vi "test4-MacroWithNonLocalSubMessages.vi"(8 "error in":errorcluster, 11 "TestCase in":refnum<class "testcase-CSMResponse.lvclass">) -> (0 "error out":errorcluster, 3 "TestCase out":refnum<class "testcase-CSMResponse.lvclass">)   [LabVIEW 2017, in "testcase-CSMResponse.lvclass"]
uses:
  testcase-CSMResponse.lvclass
  0c6454a9-3719-4e31-9ff6-45b39d38beb6.vi
  2437fcdf-222d-44ea-9250-34e015767128.vi
  src/user.lib/_NEVSTOP/Communicable State Machine(CSM)/AdvanceAPI/CSM - Get Module Attribute.vi
  <vilib>/addons/_JKI Toolkits/VI Tester/TestCase.llb/TestCase.lvclass
  src/user.lib/_NEVSTOP/Communicable State Machine(CSM)/Communicable State Machine.lvlib
  C:/Program Files (x86)/National Instruments/LabVIEW 2017/vi.lib/addons/_JKI Toolkits/VI Tester/TestCase.llb/TestCase.lvclass
panel:
  out "Loopcount":i32
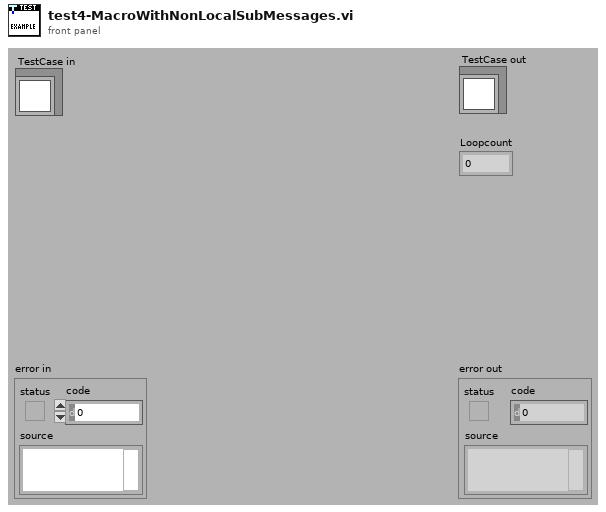
[diagram p1: front panel]
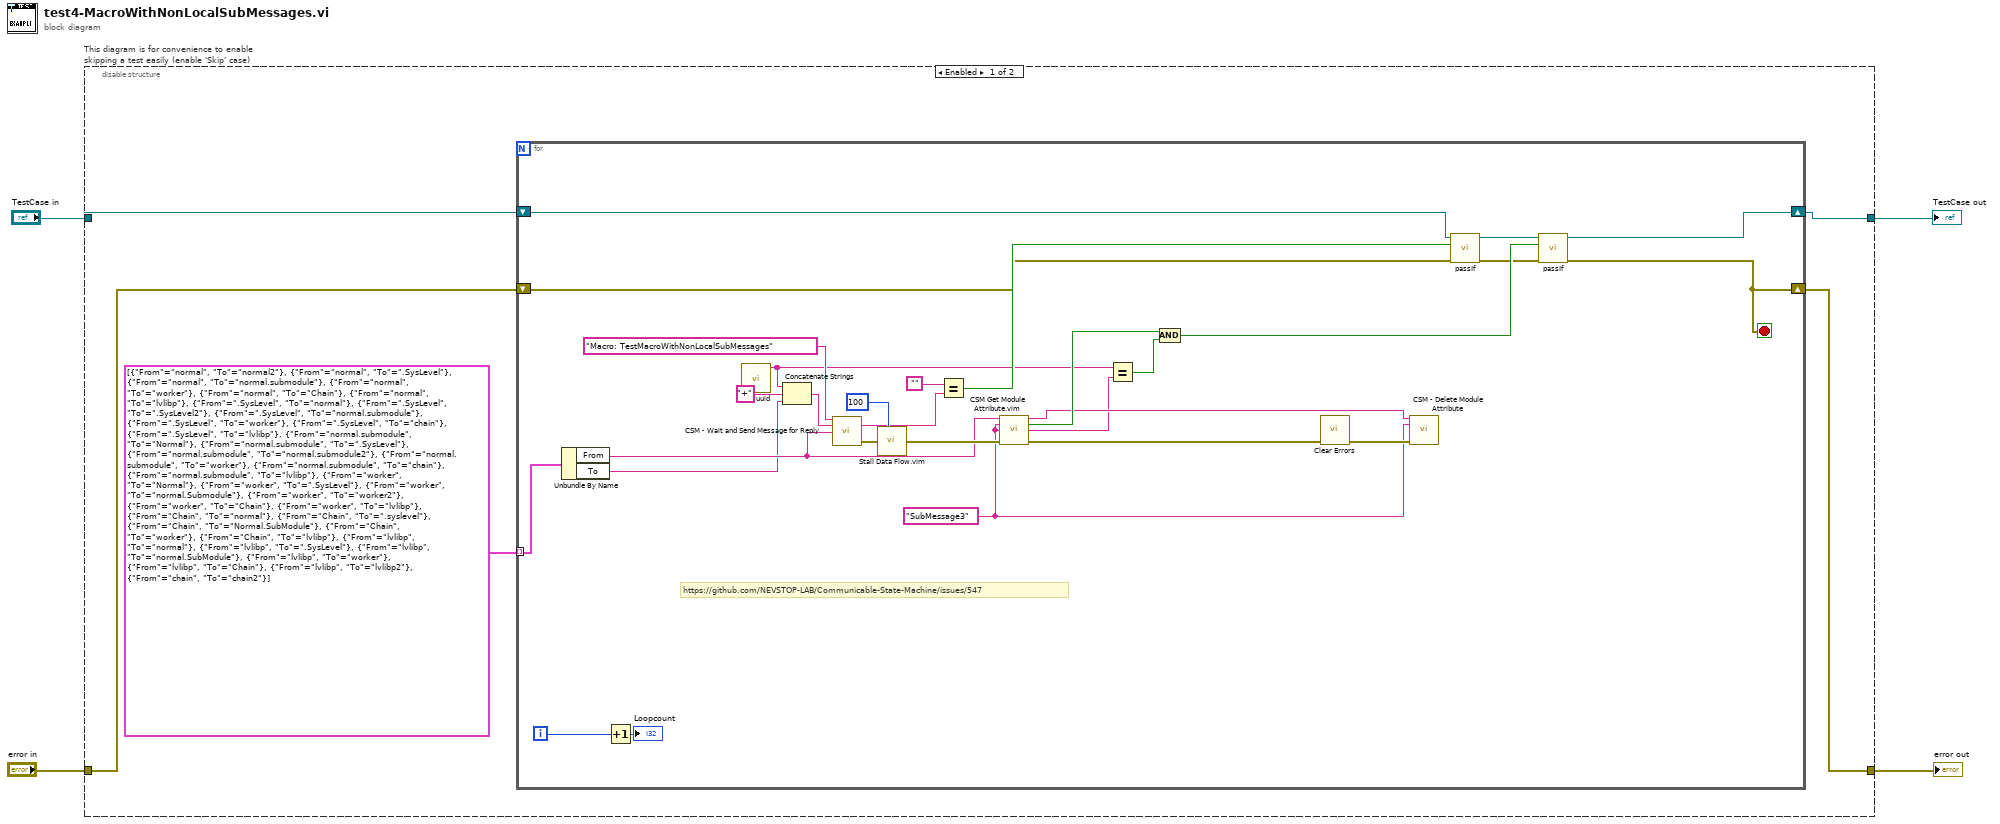
[diagram p0: block diagram]
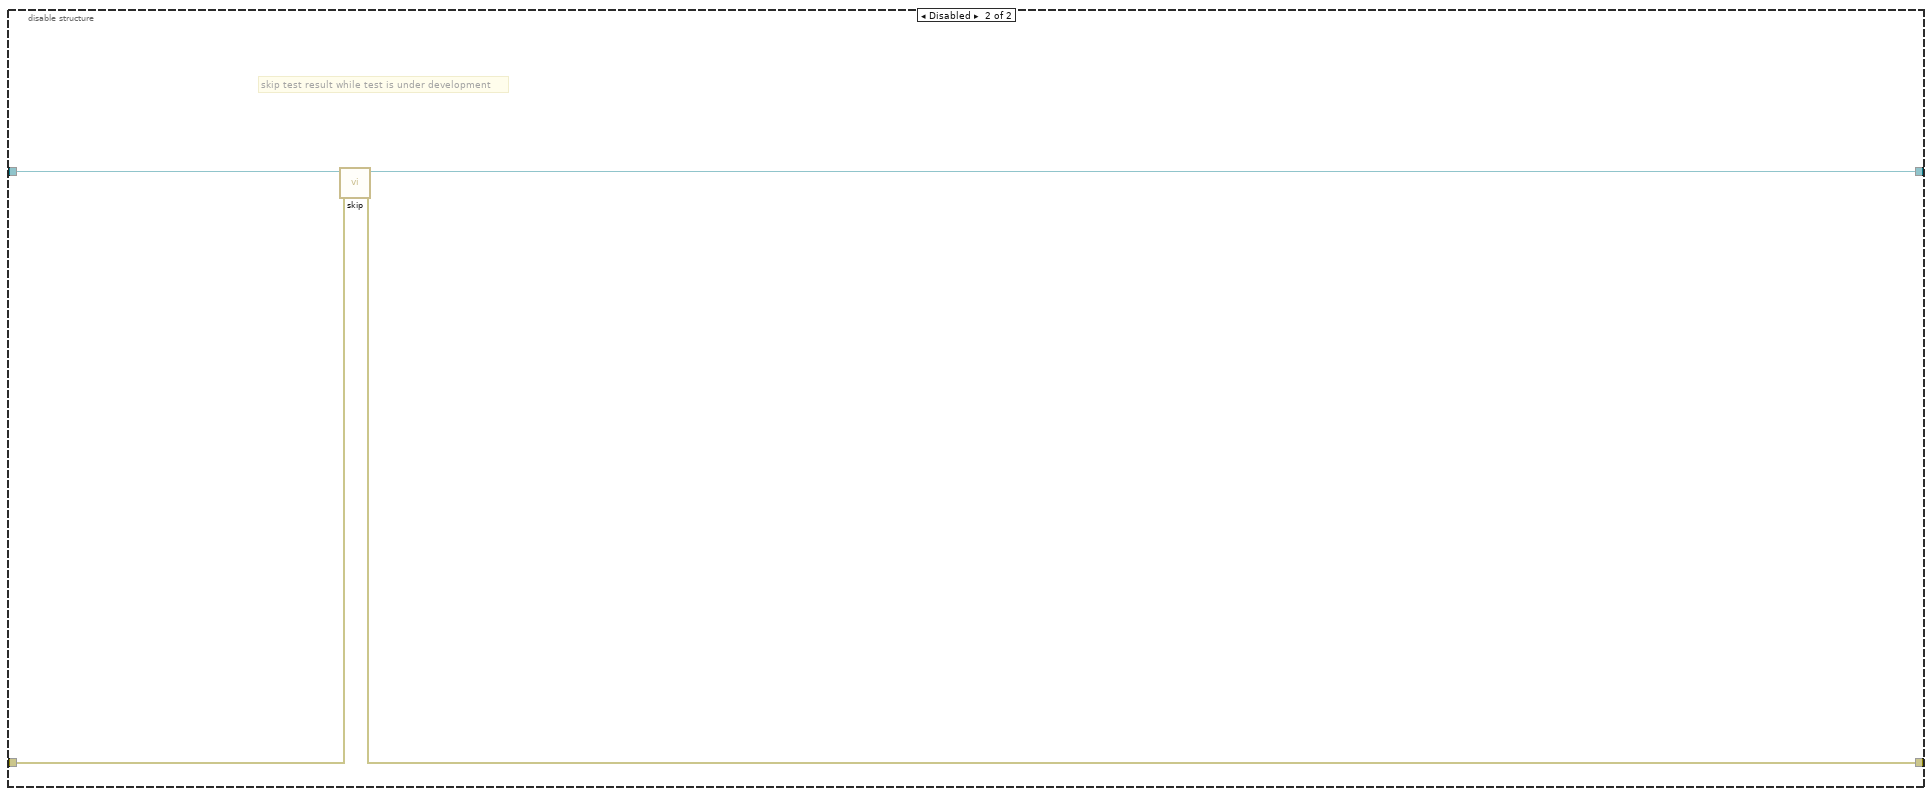
[diagram p2: hidden frame]
diagram:
  n1 = disable-structure "This diagram is for convenience to enable skipping a test easily (enable 'Skip' case)" shown="Enabled" {
    disable-tunnel: "TestCase in" -> [w9 w42]
    disable-tunnel: [w8 w40] -> w1
    disable-tunnel: [w7 w41] -> w3
    disable-tunnel: "error in" -> [w6 w39]
    frame Enabled {
      n2 = for {
        shift-right: [w25] -> w8
        shift-left: w9 -> [w20]
        shift-right: [w24] -> w7
        shift-left: w6 -> [w19]
        tunnel: cluster{"From":string, "To":string}[] [{"From"="normal", "To"="normal2"}, {"From"="normal", "To"=".SysLevel"}, {"From"="normal", "To"="normal.submodule"}, {"From"="normal", "To"="worker"}, {"From"="normal", "To"="Chain"}, {"From"="normal", "To"="lvlibp"}, {"From"=".SysLevel", "To"="normal"}, {"From"=".SysLevel", "To"=".SysLevel2"}, {"From"=".SysLevel", "To"="normal.submodule"}, {"From"=".SysLevel", "To"="worker"}, {"From"=".SysLevel", "To"="chain"}, {"From"=".SysLevel", "To"="lvlibp"}, {"From"="normal.submodule", "To"="Normal"}, {"From"="normal.submodule", "To"=".SysLevel"}, {"From"="normal.submodule", "To"="normal.submodule2"}, {"From"="normal.submodule", "To"="worker"}, {"From"="normal.submodule", "To"="chain"}, {"From"="normal.submodule", "To"="lvlibp"}, {"From"="worker", "To"="Normal"}, {"From"="worker", "To"=".SysLevel"}, {"From"="worker", "To"="normal.Submodule"}, {"From"="worker", "To"="worker2"}, {"From"="worker", "To"="Chain"}, {"From"="worker", "To"="lvlibp"}, {"From"="Chain", "To"="normal"}, {"From"="Chain", "To"=".syslevel"}, {"From"="Chain", "To"="Normal.SubModule"}, {"From"="Chain", "To"="worker"}, {"From"="Chain", "To"="lvlibp"}, {"From"="lvlibp", "To"="normal"}, {"From"="lvlibp", "To"=".SysLevel"}, {"From"="lvlibp", "To"="normal.SubModule"}, {"From"="lvlibp", "To"="worker"}, {"From"="lvlibp", "To"="Chain"}, {"From"="lvlibp", "To"="lvlibp2"}, {"From"="chain", "To"="chain2"}] -> [w17] mode=indexing
        i -> [w38]
        stop <- w24 stop-if-true
        w26 = "SubMessage3" ("Attribute")
        # "https://github.com/NEVSTOP-LAB/Communicable-State-Machine/issues/547"
        n3 = Unbundle By Name(w17) -> ("From"=w16:string, "To"=w13:string)
        n4 = Increment(x=w38) -> (x+1=→"Loopcount":i32)
        n5 = call "uuid.vi"() -> ("UUID"=w15:string)  [unwired: 11 in]
        n6 = Concatenate Strings(w15, "+", w13) -> (w12:string)
        n7 = call "CSM - Wait and Send Message for Reply.vi"("State"="Macro: TestMacroWithNonLocalSubMessages", "Arguments (\"\")"=w12, "Target Module"=w16) -> ("Response"=w23:string, "error out"=w36:errorcluster)  [unwired: 10 in, 1 out]
        n8 = call "Stall Data Flow.vim"("value in"=w36, "milliseconds to wait"=u32 100) -> ("value out"=w34:errorcluster)  [unwired: 1 out]
        n9 = Equal?(x="", y=w23) -> (x = y?=w22:bool)
        n10 = call "CSM Get Module Attribute.vim"("CSM Name"=w16, "Attribute"=w26, "Default Value (Empty Variant)"=w26, "Error In"=w34) -> ("CSM Name (Dup)"=w27:string, "Found"=w33:bool, "Value"=w11:string, "error out"=w29:errorcluster)  [unwired: 7 in, 1 out]
        n11 = Equal?(x=w15, y=w11) -> (x = y?=w31:bool)
        n12 = And(x=w33, y=w31) -> (x .and. y?=w30:bool)
        n13 = call <vilib>:"Clear Errors.vi"("error in (no error)"=w29) -> ("error out"=w28:errorcluster)  [unwired: 5 in, 1 out]
        n14 = call "CSM - Delete Module Attribute.vi"("CSM Name"=w27, "Attribute"=w26, "Error In"=w28) -> ()  [unwired: 9 in, 4 out]
        n15 = call-dynamic "passIf.vi"("error in (no error)"=w19, "pass"=w22, "TestCase in"=w20) -> ("error out"=w18:errorcluster, "TestCase out"=w21:refnum<class "testcase-CSMResponse.lvclass">)  [unwired: 7 in]
        n16 = call-dynamic "passIf.vi"("error in (no error)"=w18, "pass"=w30, "TestCase in"=w21) -> ("error out"=w24:errorcluster, "TestCase out"=w25:refnum<class "testcase-CSMResponse.lvclass">)  [unwired: 7 in]
      }
    }
    frame Disabled {
      # "skip test result while test is under development"
      n17 = call <vilib>:"skip.vi"("error in (no error)"=w39, "TestCase in"=w42) -> ("error out"=w41:errorcluster, "TestCase out"=w40:refnum<class "testcase-CSMResponse.lvclass">)  [unwired: 8 in]
    }
  }
  "error out" <- w3
  "TestCase out" <- w1
